vi "Compile Event Measure 1.1 Data.vi"(8 "error in (no error)":errorcluster, 11 "Device Item Ref in":T3 format="%.0x") -> (0 "error out":errorcluster, 2 "Event Timing Measures":T1[](array[typedef]), 3 "Device Item Ref out":T3 format="%.0x")   [LabVIEW 2013, in "Engine Simulation Toolkit System Explorer.lvlib"]
uses:
  Engine Simulation Toolkit System Explorer.lvlib
  <vilib>/NI Veristand/Custom Device API/Custom Device Item Ref.ctl
  Shared/1.1 Event Timing Measure Engine Data.ctl
  Shared/1.0 Event Timing Measure FIFO Idxs.ctl
  <vilib>/NI Veristand/Custom Device Tools/Custom Device Utility Library/Search Direction.ctl
  Polarity.ctl
  Shared/Constants and GUIDs.vi
  <vilib>/NI Veristand/Custom Device Tools/Custom Device Utility Library/NI VeriStand - Search for Item by GUID.vi
  <vilib>/NI Veristand/Custom Device Tools/Custom Device Utility Library/NI VeriStand - Search for All Items by GUID.vi
  Shared/Engine Simulation Toolkit Shared.lvlib
  <vilib>/NI Veristand/Custom Device Tools/Custom Device Utility Library/Custom Device Utility Library.lvlib
  <vilib>/NI Veristand/Custom Device API/Custom Device API.lvlib
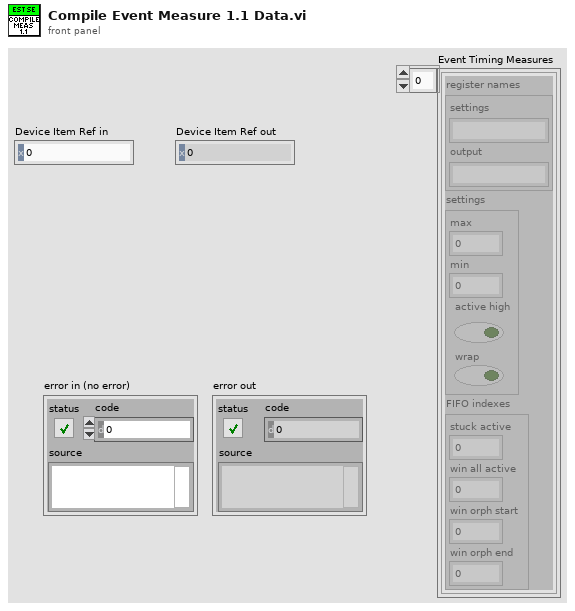
[diagram p1: front panel]
types:
  T1 = typedef "Engine Simulation Toolkit Shared.lvlib/1.1 Event Timing Measure Engine Data.ctl" = cluster{"register names":cluster{"settings":string, "output":string}, "settings":cluster{"max":u16, "min":u16, "active high":bool, "wrap":bool}, "FIFO indexes":T2}
  T2 = typedef "Engine Simulation Toolkit Shared.lvlib/1.0 Event Timing Measure FIFO Idxs.ctl" = cluster{"stuck active":i32, "win all active":i32, "win orph start":i32, "win orph end":i32}
  T3 = typedef "Custom Device API.lvlib/Custom Device Item Ref.ctl" = u64
  T4 = typedef "Custom Device Utility Library.lvlib/Search Direction.ctl" = enum16{"Down", "Up"}
  T5 = typedef "Engine Simulation Toolkit Shared.lvlib/Channel.ctl" = cluster{"Name":string, "Units":string, "Default":dbl, "Description":string}
  T6 = typedef "Custom Device API.lvlib/Custom Device Item Info.ctl" = cluster{"Name":string, "Is Channel":bool, "GUID":string, "Is Waveform":bool}
  T7 = typedef "Engine Simulation Toolkit System Explorer.lvlib/Event Timing Window.ctl" = cluster{"Name":string, "Min":dbl, "Max":dbl, "Ref":dbl}
  T8 = typedef "Engine Simulation Toolkit System Explorer.lvlib/Event Timing Measurement.ctl" = cluster{"Name":string, "Bitfile name":string, "Window":string, "Polarity":T9}
  T9 = typedef "Engine Simulation Toolkit System Explorer.lvlib/Polarity.ctl" = enum16{"Active low", "Active high"}
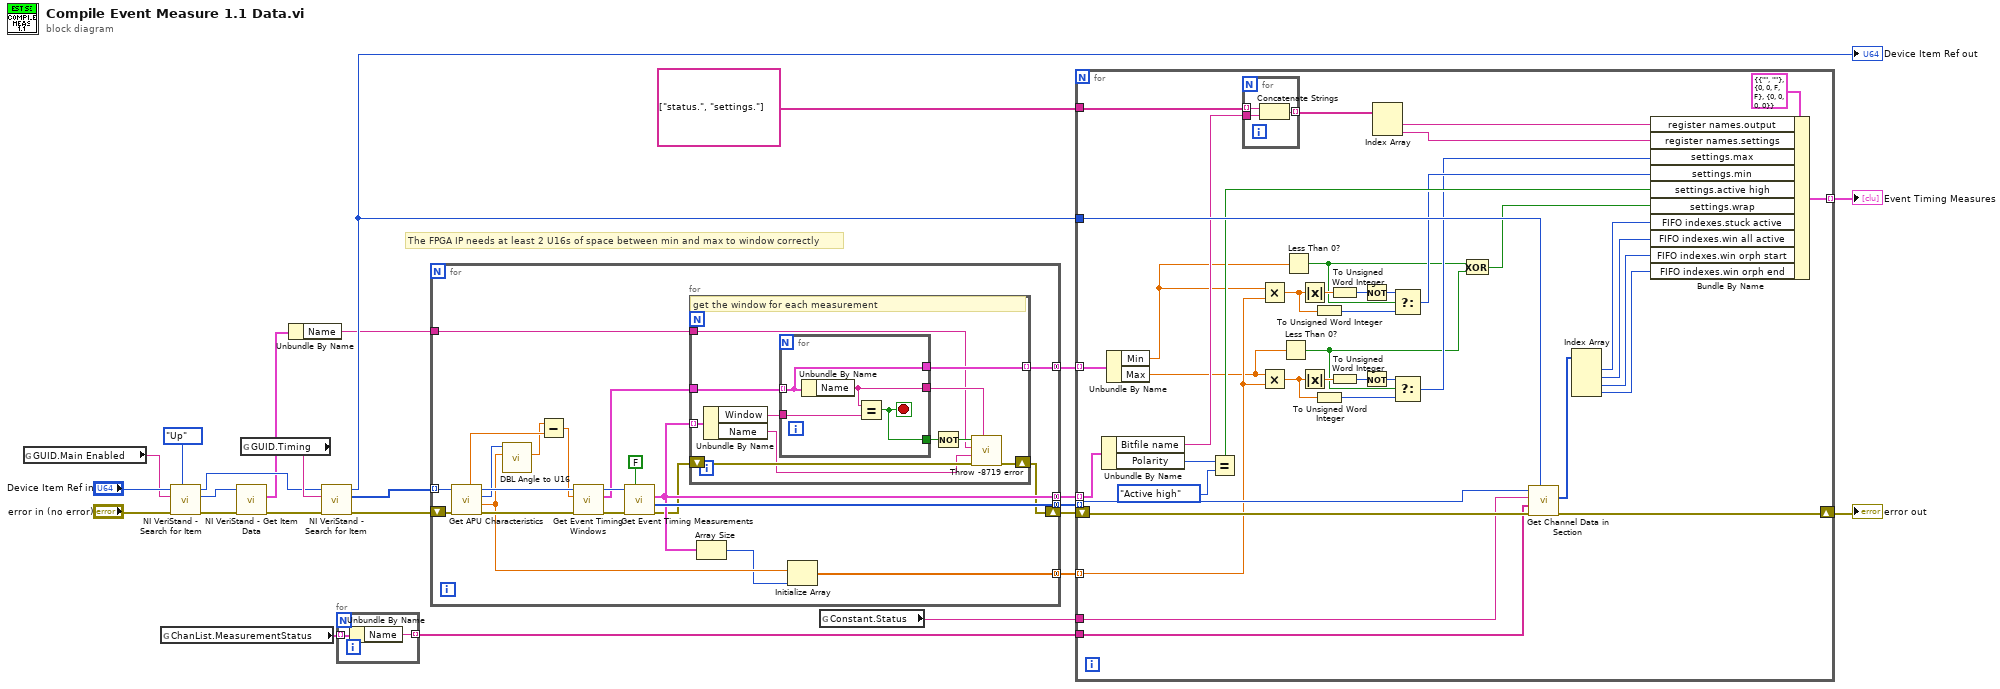
[diagram p0: block diagram]
diagram:
  # "The FPGA IP needs at least 2 U16s of space between min and max to window correctly"
  n1 = global read "Constants and GUIDs.vi" "GUID.Main Enabled"() -> (w7:string)
  n2 = global read "Constants and GUIDs.vi" "ChanList.MeasurementStatus"() -> (w19:T5[])
  n3 = call-poly <vilib>:"NI VeriStand - Search for Item.vi"("Direction (Down)"=Search_Direction."Up", "error in"="error in (no error)", "Item GUID"=w7, "Section Ref in"="Device Item Ref in") -> ("error out"=w9:errorcluster, "Item Ref"=w4:T3, "Section Ref out"=w3:T3)  [unwired: 4 in, 1 out]
  n4 = call <vilib>:"NI VeriStand - Get Item Data.vi"("error in (no error)"=w9, "Item Ref in"=w4) -> ("error out"=w5:errorcluster, "Item Info"=w2:T6)  [unwired: 6 in, 2 out]
  n5 = global read "Constants and GUIDs.vi" "GUID.Timing"() -> (w17:string)
  n6 = Unbundle By Name(w2) -> ("Name"=w1:string)
  n7 = call-poly <vilib>:"NI VeriStand - Search for Item.vi"("error in"=w5, "Item GUID"=w17, "Section Ref in"=w3) -> ("error out"=w24:errorcluster, "Item Refs"=w15:T3[], "Section Ref out"=w20:T3)  [unwired: 5 in, 1 out]
  "Device Item Ref out" <- w20
  n8 = for {
    tunnel: w19 -> [w27] mode=indexing
    tunnel: [w26] -> w18 mode=indexing
    n9 = Unbundle By Name(w27) -> ("Name"=w26:string)
  }
  n10 = for {
    tunnel: w15 -> [w43] mode=indexing
    shift-right: [w33] -> w16
    shift-left: w24 -> [w48]
    tunnel: [w39] -> w14 mode=concatenating
    tunnel: [w47] -> w13 mode=concatenating
    tunnel: [w40] -> w12 mode=concatenating
    tunnel: [w37] -> w11 mode=concatenating
    tunnel: w1 -> [w32]
    n11 = call "Get APU Characteristics.vi"("error in (no error)"=w48, "Item Ref in"=w43) -> ("error out"=w44:errorcluster, "angle to u16 scale factor"=w38:dbl, "total angle span (degrees)"=w35:u16, "Item Ref out"=w42:T3, "degrees of one u16"=w31:dbl)  [unwired: 3 in, 2 out]
    n12 = call "DBL Angle to U16.vi"("angle to u16 scale factor"=w38, "Desired angle (degrees)"=w35) -> ("Actual angle (degrees)"=w30:dbl)  [unwired: 8 in, 1 out]
    n13 = Subtract(x=w30, y=w31) -> (x-y=w29:dbl)
    n14 = call "Get Event Timing Windows.vi"("error in (no error)"=w44, "Max engine angle"=w29, "Item Ref in"=w42) -> ("error out"=w46:errorcluster, "Windows"=w41:T7[], "Item Ref out"=w45:T3)  [unwired: 6 in]
    n15 = call "Get Event Timing Measurements.vi"("return not-added measurements (T)"=FALSE, "error in (no error)"=w46, "Item Ref in"=w45) -> ("error out"=w34:errorcluster, "measurements refs"=w47:T3[], "measurements"=w39:T8[])  [unwired: 4 in, 2 out]
    n16 = for {
      tunnel: w39 -> [w59] mode=indexing
      tunnel: w41 -> [w58]
      tunnel: [w56] -> w40 mode=indexing
      shift-right: [w52] -> w33
      shift-left: w34 -> [w51]
      tunnel: w32 -> [w49]
      # "get the window for each measurement"
      n17 = Unbundle By Name(w59) -> ("Window"=w57:string, "Name"=w50:string)
      n18 = for {
        tunnel: w58 -> [w62] mode=indexing
        tunnel: w57 -> [w63]
        tunnel: [w62] -> w56
        tunnel: [w61] -> w55
        tunnel: [w60] -> w53
        stop <- w61 stop-if-true
        n19 = Unbundle By Name(w62) -> ("Name"=w60:string)
        n20 = Equal?(x=w60, y=w63) -> (x = y?=w61:bool)
      }
      n21 = Not(x=w55) -> (.not. x?=w54:bool)
      n22 = call "Throw -8719 error.vi"("window name"=w53, "error in (no error)"=w51, "measurement name"=w50, "Custom device name"=w49, "Error"=w54) -> ("error out"=w52:errorcluster)  [unwired: 6 in]
    }
    n23 = Array Size(array=w39) -> (size(s)=w36:i32)
    n24 = Initialize Array(w38, w36) -> (w37:dbl[])
  }
  n25 = global read "Constants and GUIDs.vi" "Constant.Status"() -> (w10:string)
  n26 = for {
    shift-right: [w97] -> w22
    shift-left: w16 -> [w100]
    tunnel: string[] ["status.", "settings."] -> [w104]
    tunnel: w18 -> [w98]
    tunnel: [w102] -> w21 mode=indexing
    tunnel: w20 -> [w99]
    tunnel: w14 -> [w88] mode=indexing
    tunnel: w13 -> [w76] mode=indexing
    tunnel: w12 -> [w89] mode=indexing
    tunnel: w11 -> [w70] mode=indexing
    tunnel: w10 -> [w75]
    n27 = Unbundle By Name(w88) -> ("Bitfile name"=w87:string, "Polarity"=w86:T9)
    n28 = Unbundle By Name(w89) -> ("Min"=w78:dbl, "Max"=w67:dbl)
    n29 = Equal?(x=w86, y=Polarity."Active high") -> (x = y?=w84:bool)
    n30 = for {
      tunnel: w104 -> [w107] mode=indexing
      tunnel: [w106] -> w101 mode=indexing
      tunnel: w87 -> [w105]
      n31 = Concatenate Strings(w107, w105) -> (w106:string)
    }
    n32 = Multiply(x=w78, y=w70) -> (x*y=w79:dbl)
    n33 = Multiply(x=w67, y=w70) -> (x*y=w68:dbl)
    n34 = Less Than 0?(x=w67) -> (x < 0?=w65:bool)
    n35 = Less Than 0?(x=w78) -> (x < 0?=w66:bool)
    n36 = Absolute Value(x=w79) -> (abs(x)=w81:dbl)
    n37 = Absolute Value(x=w68) -> (abs(x)=w73:dbl)
    n38 = To Unsigned Word Integer(number=w79) -> (unsigned 16bit integer=w83:u16)
    n39 = To Unsigned Word Integer(number=w68) -> (unsigned 16bit integer=w71:u16)
    n40 = To Unsigned Word Integer(number=w81) -> (unsigned 16bit integer=w80:u16)
    n41 = To Unsigned Word Integer(number=w73) -> (unsigned 16bit integer=w74:u16)
    n42 = Not(x=w80) -> (.not. x?=w82:u16)
    n43 = Not(x=w74) -> (.not. x?=w72:u16)
    n44 = Index Array(array=w101) -> (element #1=w95:string, element #2=w94:string)  [unwired: 2 in]
    n45 = Select(t=w82, s=w66, f=w83) -> (s? t:f=w77:u16)
    n46 = Select(t=w72, s=w65, f=w71) -> (s? t:f=w69:u16)
    n47 = Exclusive Or(1:w65, 2:w66) -> (0:w64:bool)
    n48 = call "Get Channel Data in Section.vi"("Custom device ref"=w99, "error in (no error)"=w100, "Channels"=w98, "Section (\"\":none)"=w75, "Item Ref in"=w76) -> ("error out"=w97:errorcluster, "FIFO indexes"=w96:i32[])  [unwired: 2 in, 3 out]
    n49 = Index Array(array=w96) -> (element #1=w93:i32, element #2=w92:i32, element #3=w91:i32, element #4=w90:i32)  [unwired: 4 in]
    n50 = Bundle By Name(cluster=T1 {"register names"={"settings"="", "output"=""}, "settings"={"max"=0, "min"=0, "active high"=FALSE, "wrap"=FALSE}, "FIFO indexes"={"stuck active"=0, "win all active"=0, "win orph start"=0, "win orph end"=0}} ("1.0.0 Event Timing Measure"), "register names.output"=w95, "register names.settings"=w94, "settings.max"=w69, "settings.min"=w77, "settings.active high"=w84, "settings.wrap"=w64, "FIFO indexes.stuck active"=w93, "FIFO indexes.win all active"=w92, "FIFO indexes.win orph start"=w91, "FIFO indexes.win orph end"=w90) -> (w102:T1)
  }
  "error out" <- w22
  "Event Timing Measures" <- w21
